vi "Close.vi"(8 "error in (no error)":errorcluster, 11 "All Queue in":T1) -> (0 "error out":errorcluster)   [LabVIEW 2015, in "UndoLibrary.lvlib"]
doc: "This VI destroys the references to store the values of the control."
uses:
  UndoLibrary.lvlib
  Controls/cluster_All Queue.ctl
  Controls/cluster_Control Value.ctl
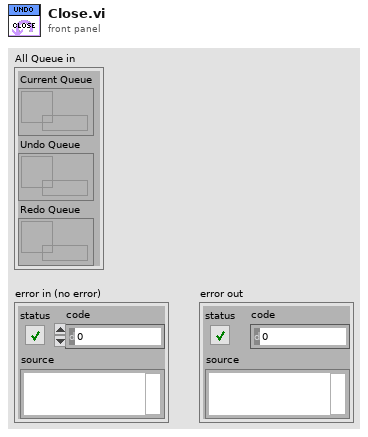
[diagram p1: front panel]
types:
  T1 = typedef "UndoLibrary.lvlib/cluster_All Queue.ctl" = cluster{"Current Queue":refnum<queue>, "Undo Queue":refnum<queue>, "Redo Queue":refnum<queue>}
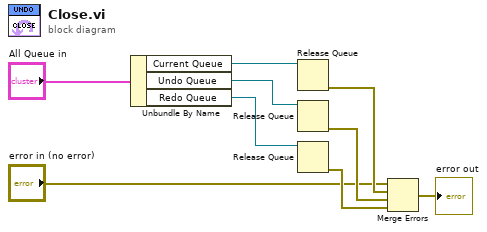
[diagram p0: block diagram]
diagram:
  n1 = Unbundle By Name("All Queue in") -> ("Current Queue"=w3:refnum<queue>, "Undo Queue"=w4:refnum<queue>, "Redo Queue"=w5:refnum<queue>)
  n2 = Release Queue(queue=w3) -> (error out=w8:errorcluster)  [unwired: 2 in, 2 out]
  n3 = Release Queue(queue=w4) -> (error out=w7:errorcluster)  [unwired: 2 in, 2 out]
  n4 = Release Queue(queue=w5) -> (error out=w6:errorcluster)  [unwired: 2 in, 2 out]
  n5 = Merge Errors("error in (no error)", w8, w7, w6) -> (→"error out":errorcluster)
